vi "LDA_IP_DataTranslation.vi"() -> ()   [LabVIEW 2011]
uses:
  Globals/Meas_global.vi
  Data_Translation/DataTranslation_global.vi
  Globals/LDA_meas_global_1.vi
  PWA/PWAtasksGLOBAL.vi
  <userlib>/LV-Link3/PolySubVIs/DtCreateAinChan.vi
  <userlib>/LV-Link3/PolySubVIs/DtOLTimingSetInput.vi
  <userlib>/LV-Link3/PolySubVIs/DtOLTriggerDigital.vi
  Globals/LDA_meas_global_2.vi
  <userlib>/LV-Link3/PolySubVIs/DtOLReadMultiple2D.vi
panel:
  out "error out":errorcluster
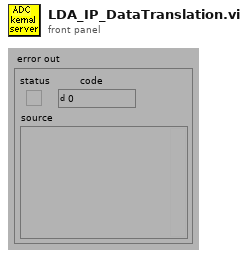
[diagram p1: front panel]
types:
  T1 = typedef "Ch_and_Spans.ctl" = cluster{"high limit (10V)":sgl, "low limit (-10V)":sgl, "Ch No":i16, "Var name":string, "Use Latest Calib":bool}
  T2 = typedef "Trigger_Mode.ctl" = enum16{"Free Running", "Start on Trigger", "Trigger Every Block", "Trigger Every Sample"}
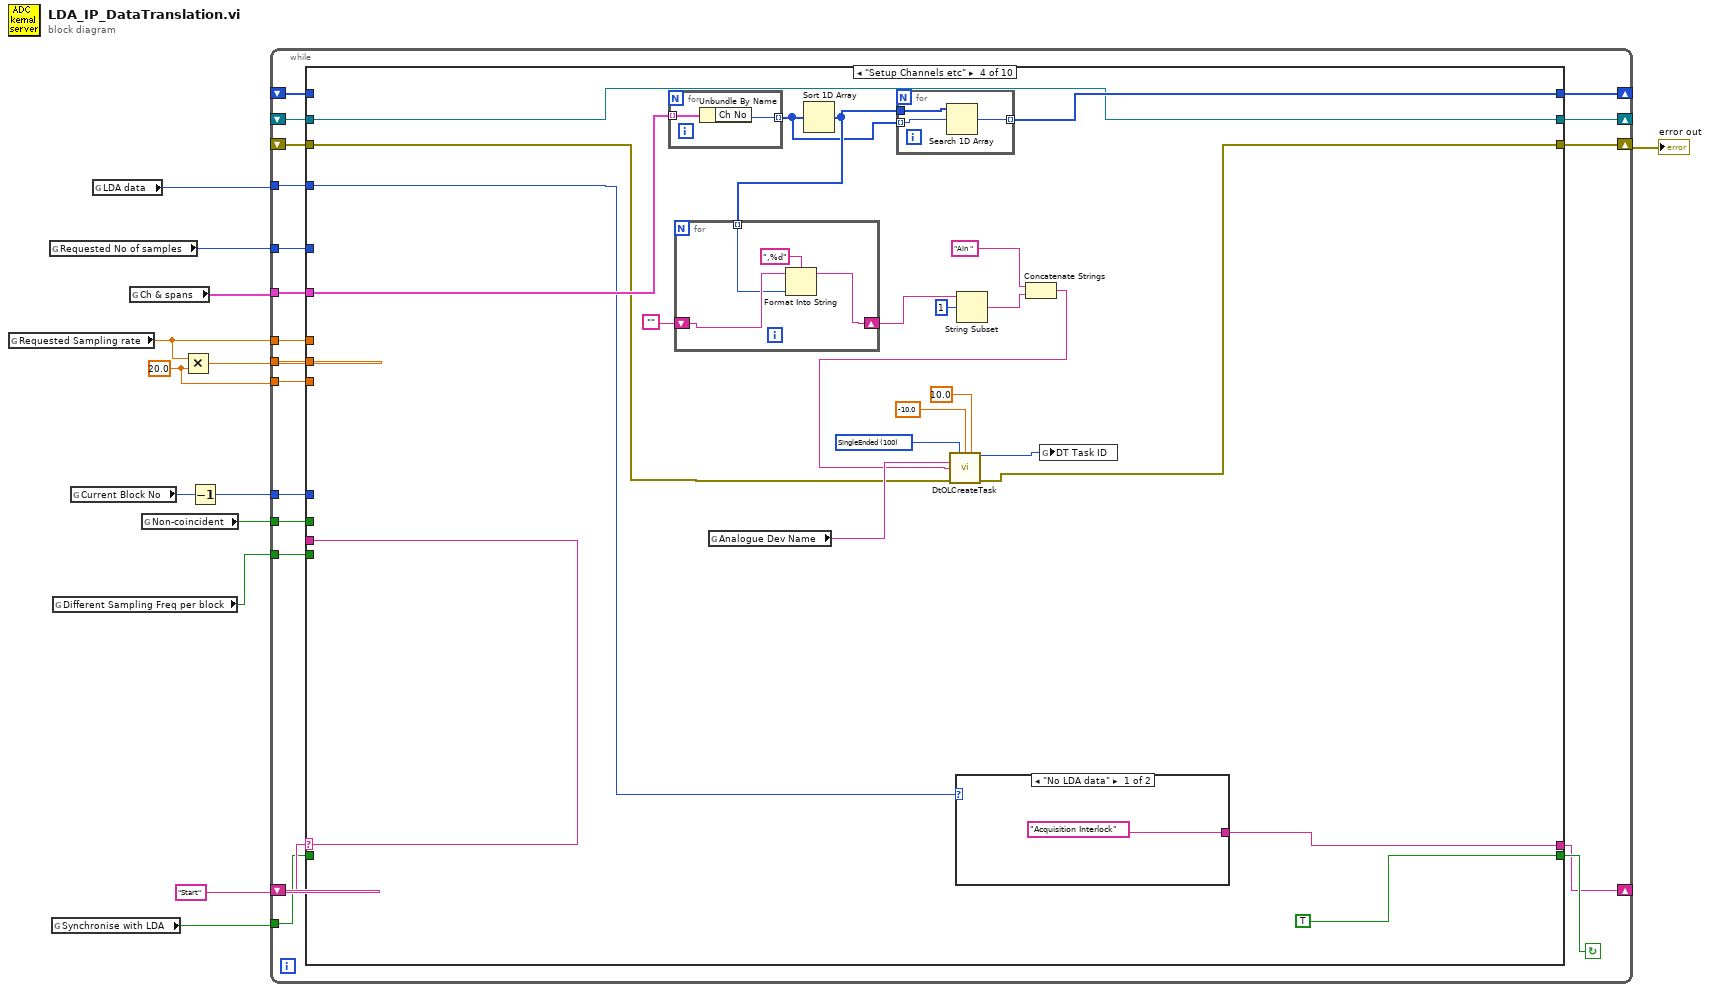
[diagram p0: block diagram]
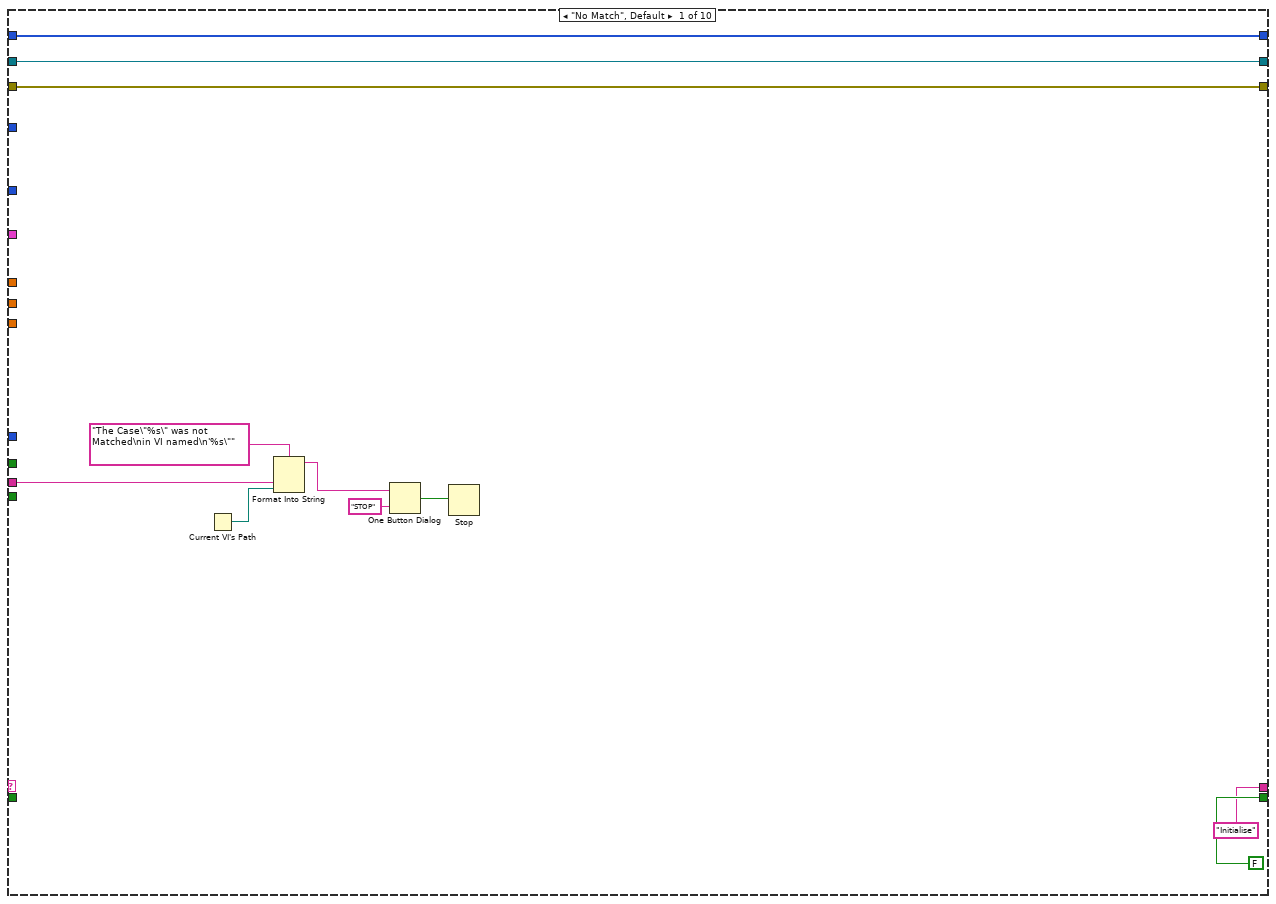
[diagram p2: hidden frame]
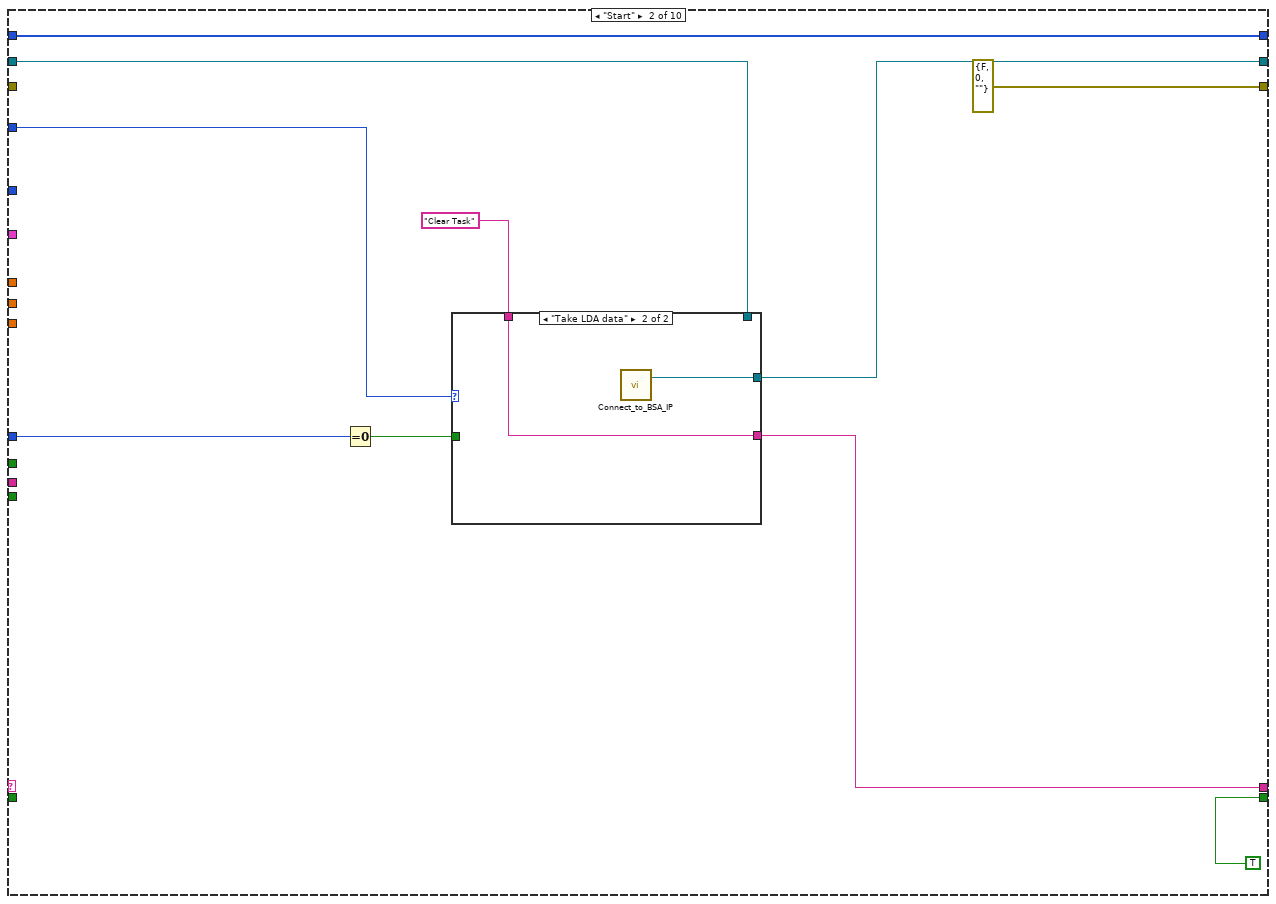
[diagram p3: hidden frame]
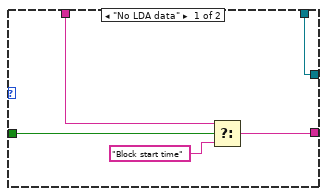
[diagram p4: hidden frame]
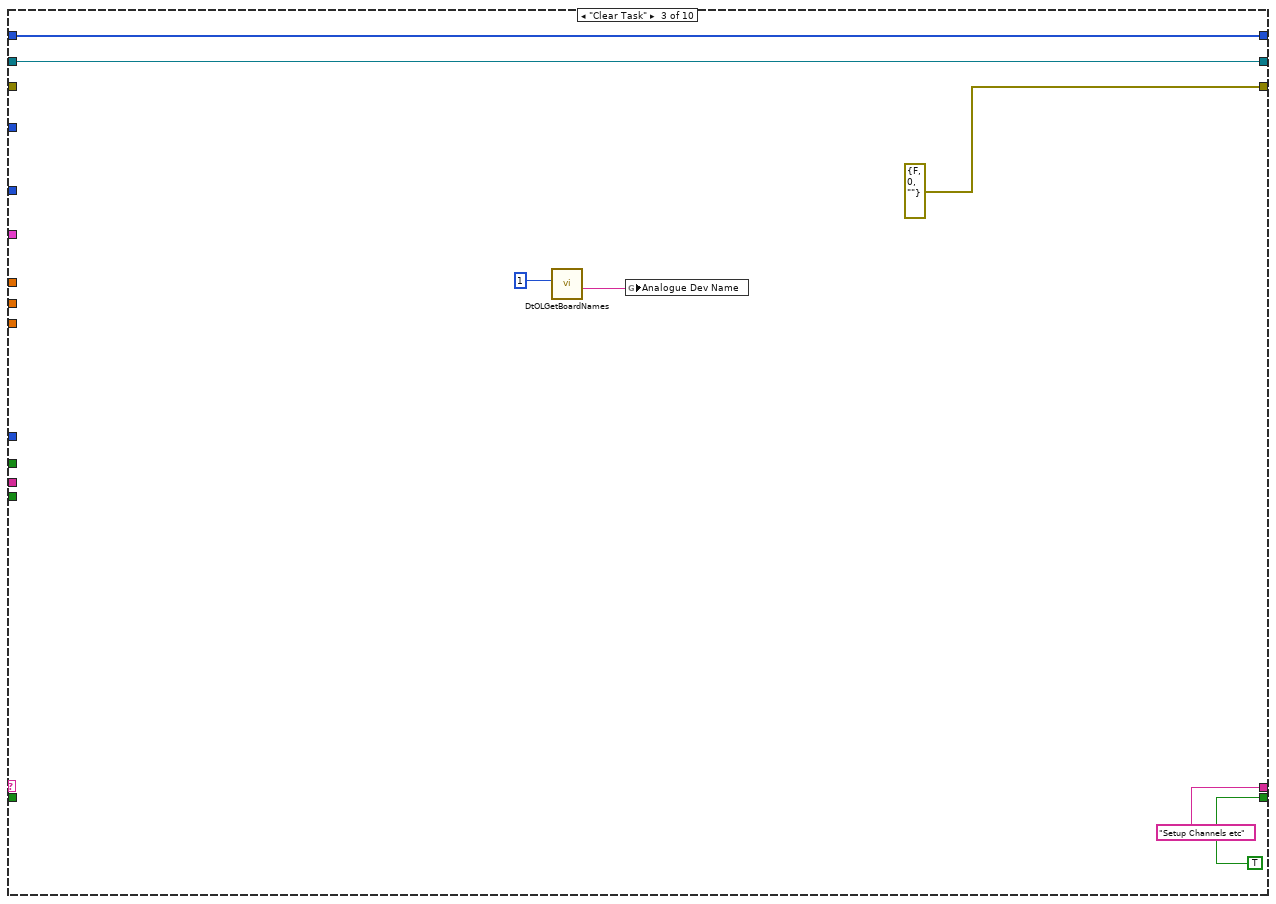
[diagram p5: hidden frame]
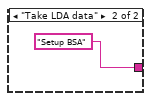
[diagram p6: hidden frame]
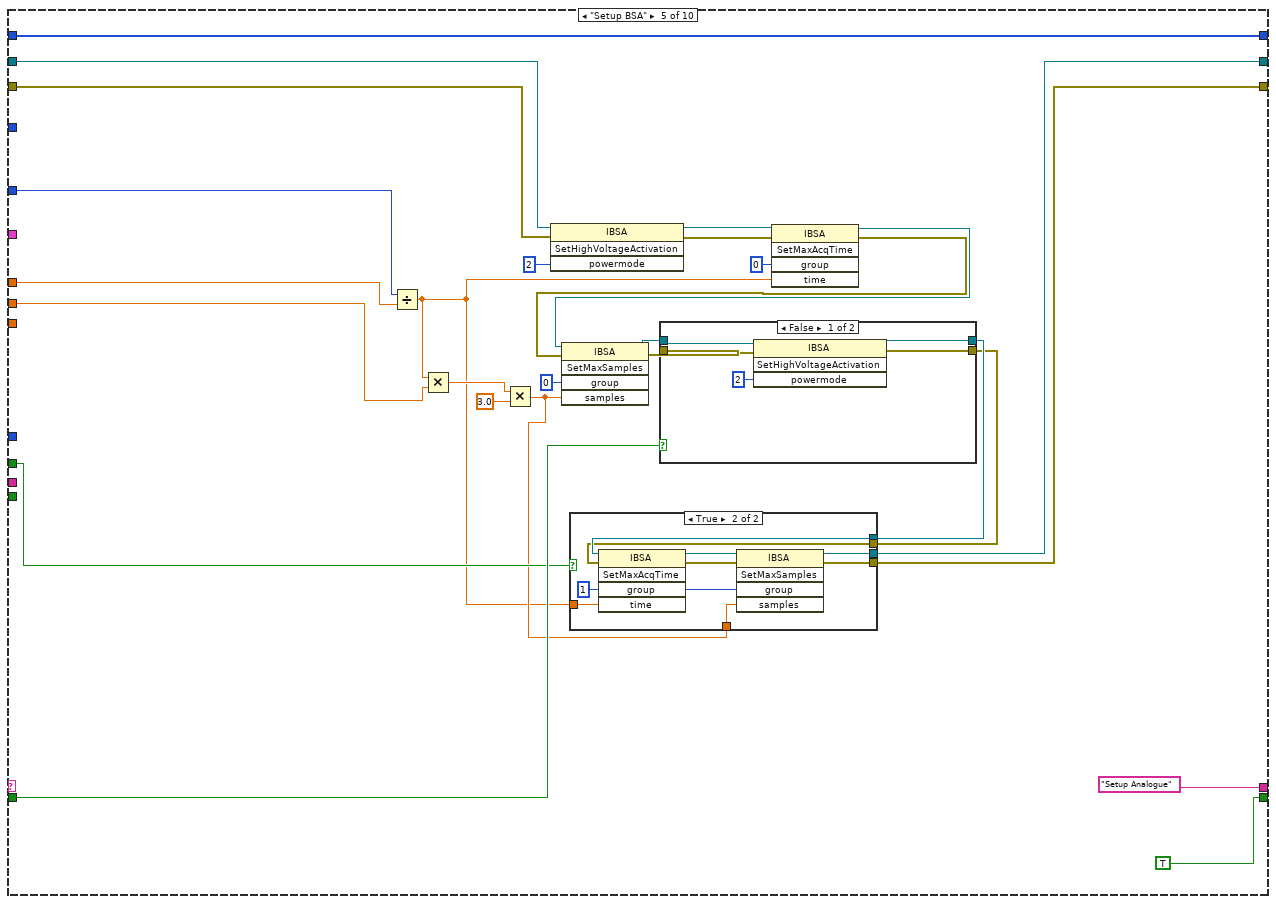
[diagram p7: hidden frame]
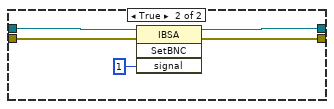
[diagram p9: hidden frame]
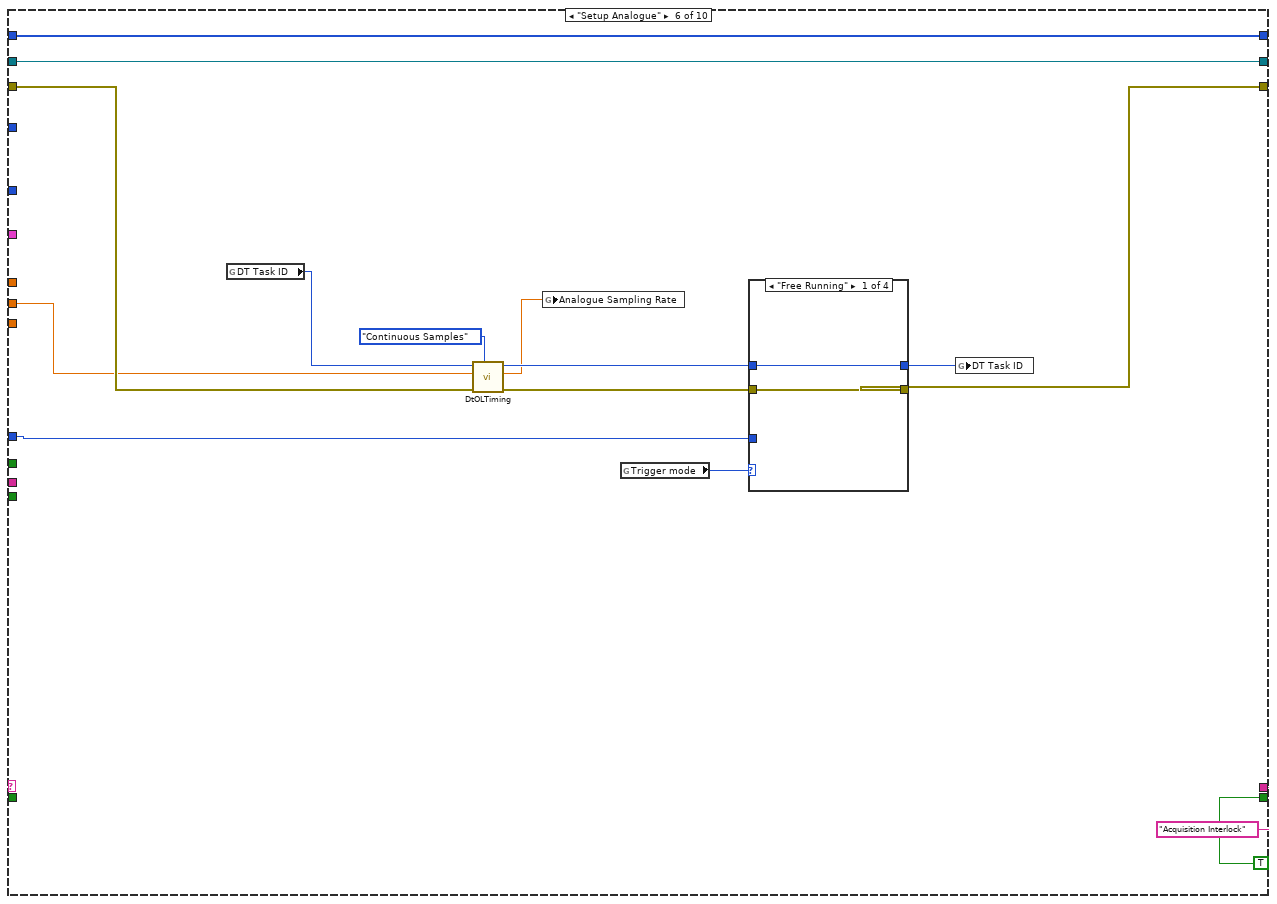
[diagram p10: hidden frame]
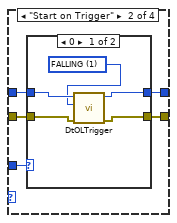
[diagram p11: hidden frame]
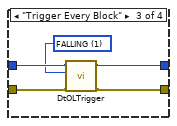
[diagram p13: hidden frame]
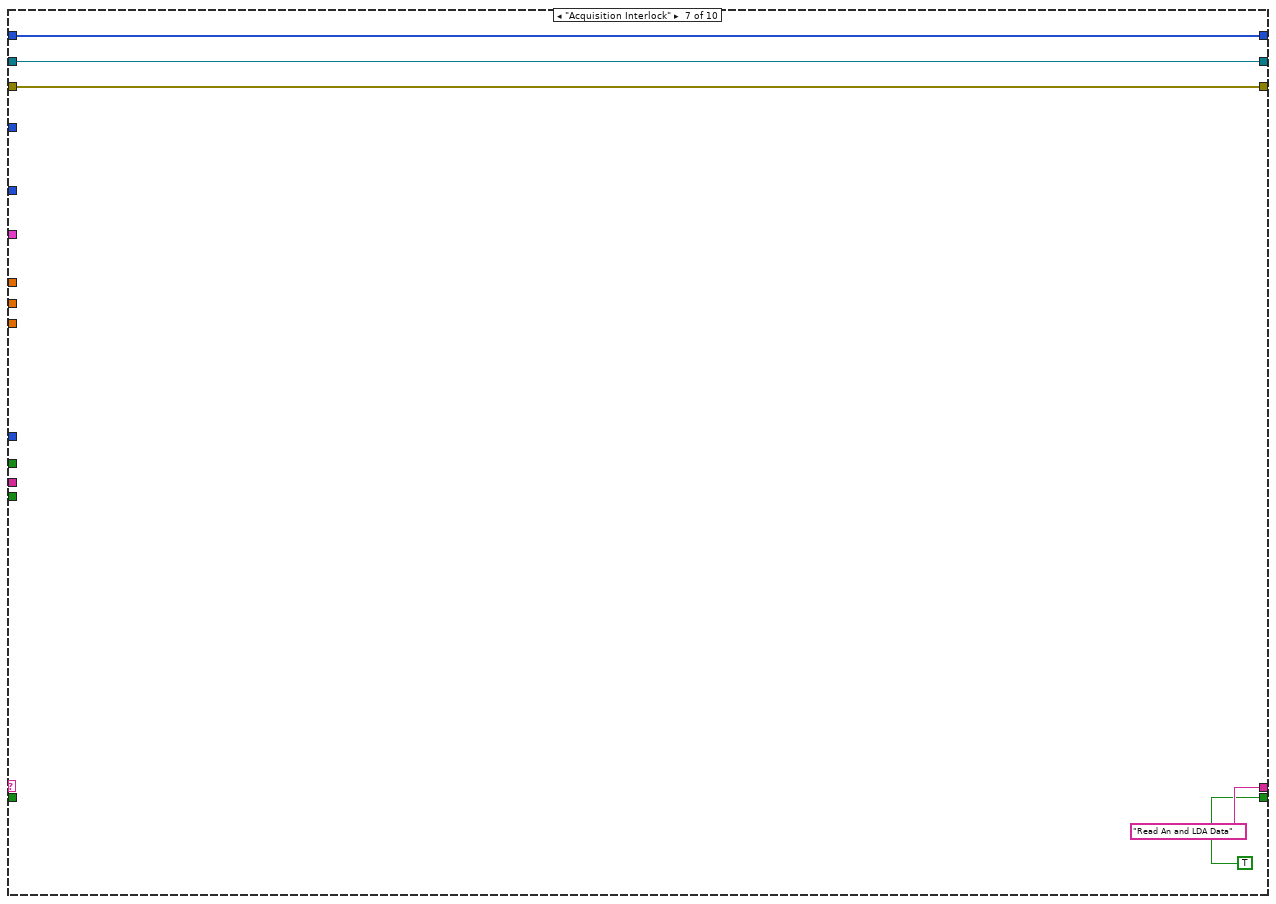
[diagram p15: hidden frame]
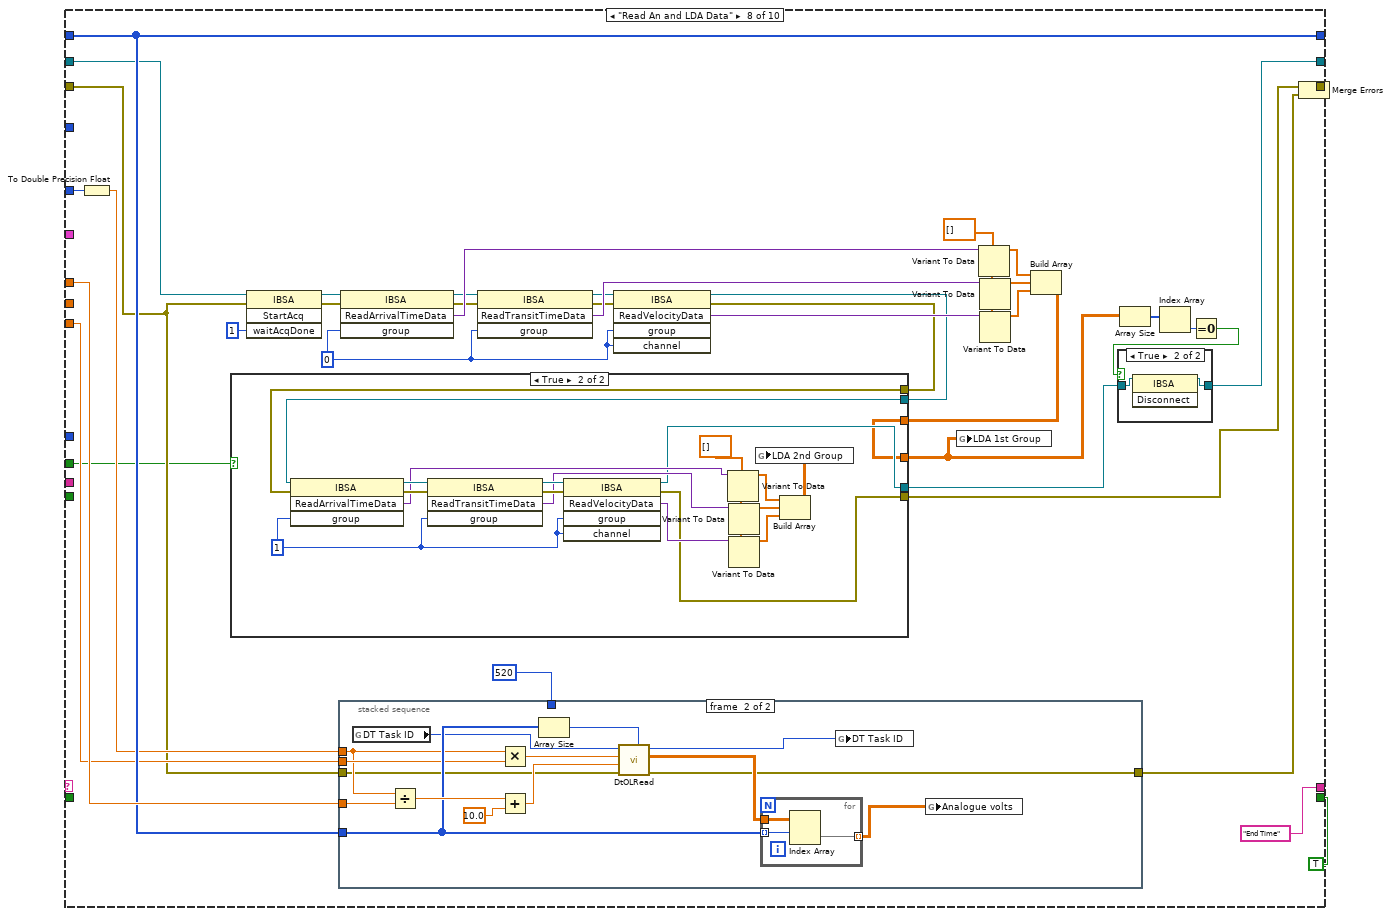
[diagram p16: hidden frame]
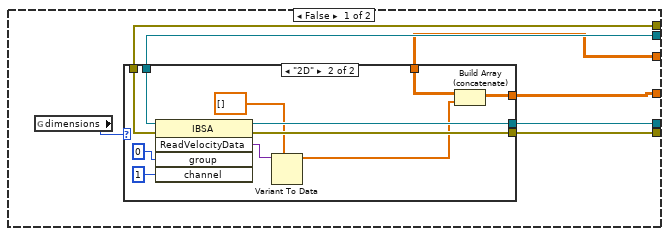
[diagram p17: hidden frame]
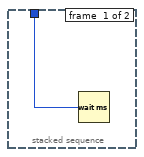
[diagram p20: hidden frame]
diagram:
  w8 = 20.0 ("y")
  n1 = global read "Meas_global.vi" "Requested Sampling rate"() -> (w2:dbl)
  n2 = global read "Meas_global.vi" "Requested No of samples"() -> (w1:i32)
  n3 = global read "Meas_global.vi" "Synchronise with LDA"() -> (w10:bool)
  n4 = global read "DataTranslation_global.vi" "Different Sampling Freq per block"() -> (w7:bool)
  n5 = global read "Meas_global.vi" "Current Block No"() -> (w5:i32)
  n6 = global read "Meas_global.vi" "LDA data"() -> (w11:enum16{"No LDA data", "Take LDA data"})
  n7 = global read "Meas_global.vi" "Ch & spans"() -> (w3:T1[])
  n8 = global read "LDA_meas_global_1.vi" "Non-coincident"() -> (w6:bool)
  n9 = Multiply(x=w2, y=w8) -> (x*y=w9:dbl)
  n10 = Decrement(x=w5) -> (x-1=w4:i32)
  n11 = while {
    shift-left: "Start" -> [w30]
    shift-right: [w31] -> _
    shift-right: [w24] -> w12
    shift-left: _ -> [w29]
    tunnel: w2 -> [w28]
    tunnel: w1 -> [w27]
    tunnel: w4 -> [w26]
    tunnel: w3 -> [w25]
    shift-right: [w23] -> _
    shift-left: _ -> [w22]
    tunnel: w11 -> [w21]
    shift-right: [w20] -> _
    shift-left: _ -> [w19]
    tunnel: w10 -> [w18]
    tunnel: w9 -> [w17]
    tunnel: w8 -> [w16]
    tunnel: w7 -> [w15]
    tunnel: w6 -> [w14]
    stop <- w32 continue-if-true
    n12 = case shown="\"Setup Channels etc\"" w30 {
      tunnel: [FALSE TRUE TRUE TRUE TRUE TRUE TRUE TRUE FALSE FALSE] -> w32
      tunnel: ["Initialise" w50 "Setup Channels etc" w88 "Setup Analogue" "Acquisition Interlock" "Read An and LDA Data" "End Time" "End" ("f") "End" ("f")] -> w31
      tunnel: w30 -> [w38 _ _ _ _ _ _ _ _ _]
      tunnel: [w35 errorcluster {"status"=FALSE, "code"=0, "source"=""} ("error out") errorcluster {"status"=FALSE, "code"=0, "source"=""} ("error out") w68 w100 w152 w187 w221 w296 w309] -> w24
      tunnel: w29 -> [w35 _ _ w69 w116 w159 w187 w214 w297 w309]
      tunnel: w28 -> [_ _ _ _ w113 _ _ w224 _ _]
      tunnel: w27 -> [_ _ _ _ w115 _ _ w217 _ _]
      tunnel: w26 -> [_ w52 _ _ _ w155 _ _ _ _]
      tunnel: w25 -> [_ _ _ w81 _ _ _ _ _ _]
      tunnel: [w34 w48 w65 w78 w112 w154 w185 w219 w300 w308] -> w23
      tunnel: w22 -> [w34 w48 w65 _ w112 w154 w185 w219 w300 w308]
      tunnel: w21 -> [_ w47 _ w76 _ _ _ _ w291 _]
      tunnel: [w33 w45 w64 w77 w101 w162 w184 w220 w299 w307] -> w20
      tunnel: w19 -> [w33 w44 w64 w77 w117 w162 w184 w215 w299 w307]
      tunnel: w18 -> [_ _ _ _ w114 _ _ _ _ _]
      tunnel: w17 -> [_ _ _ _ w109 w157 _ _ _ _]
      tunnel: w16 -> [_ _ _ _ _ _ _ w218 _ _]
      tunnel: w15 -> [_ _ _ _ _ _ _ _ _ _]
      tunnel: w14 -> [_ _ _ _ w108 _ _ w213 _ _]
      frame "No Match", Default {
        n13 = Current VI's Path() -> (path=w37:path)
        n14 = Format Into String(format string="The Case\"%s\" was not Matched\nin VI named\n'%s\"" ("Format String"), w38, w37) -> (resulting string=w41:string)  [unwired: 2 in, 1 out]
        n15 = One Button Dialog(message=w41, button name ("OK")="STOP") -> (true=w39:bool)
        n16 = Stop(stop? (T)=w39) -> ()
      }
      frame "Start" {
        n17 = Equal To 0?(x=w52) -> (x = 0?=w51:bool)
        n18 = case shown="\"Take LDA data\"" w47 {
          tunnel: w51 -> [w57 _]
          tunnel: [w56 w60] -> w50
          tunnel: "Clear Task" -> [w55 w60]
          tunnel: [w54 w59] -> w45
          tunnel: w44 -> [w54 _]
          frame "No LDA data" {
            n19 = Select(t=w55, s=w57, f="Block start time") -> (s? t:f=w56:string)
          }
          frame "Take LDA data" {
            n20 = call "Connect_to_BSA_IP.vi"() -> ("BSA"=w59:refnum<k7>)  [unwired: 3 out]
          }
        }
      }
      frame "Clear Task" {
        n21 = call <userlib>:"DtOLGetBoardNames.vi"("Select Board"=u32 1) -> ("Board Name"=w61:string)  [unwired: 8 in, 2 out]
        n22 = global write "PWAtasksGLOBAL.vi" "Analogue Dev Name"(w61) -> ()
      }
      frame "Setup Channels etc" {
        w73 = 100 items=["SingleEnded"=100, "Differential"=101] ("Channel Type")
        n23 = for {
          tunnel: w81 -> [w95] mode=indexing
          tunnel: [w94] -> w79 mode=indexing
          n24 = Unbundle By Name(w95) -> ("Ch No"=w94:i16)
        }
        n25 = global read "PWAtasksGLOBAL.vi" "Analogue Dev Name"() -> (w71:string)
        n26 = Sort 1D Array(array=w79) -> (sorted array=w80:i16[])
        n27 = for {
          shift-right: [w97] -> w86
          shift-left: "" -> [w98]
          tunnel: w80 -> [w96] mode=indexing
          n28 = Format Into String(format string=",%d", initial string=w98, w96) -> (resulting string=w97:string)  [unwired: 1 in, 1 out]
        }
        n29 = for {
          tunnel: w80 -> [w93]
          tunnel: w79 -> [w92] mode=indexing
          tunnel: [w91] -> w78 mode=indexing
          n30 = Search 1D Array(1D array=w93, element=w92) -> (index of element=w91:i32)  [unwired: 1 in]
        }
        n31 = case shown="\"No LDA data\"" w76 {
          tunnel: ["Acquisition Interlock" "Setup BSA"] -> w88
          frame "No LDA data" {
          }
          frame "Take LDA data" {
          }
        }
        n32 = String Subset(string=w86, offset (0)=1) -> (substring=w83:string)  [unwired: 1 in]
        n33 = Concatenate Strings("Ain ", w83) -> (w70:string)
        n34 = call-poly <userlib>:"DtOLCreateTask.vi"("Channel Type"=w73, "Range Min"=-10.0, "Range Max"=10.0, "Board Name"=w71, "Channel"=w70, "error in (no error)"=w69) -> ("Task out"=w72:i32, "error out"=w68:errorcluster)  [unwired: 7 in, 1 out]
        n35 = global write "DataTranslation_global.vi" "DT Task ID"(w72) -> ()
      }
      frame "Setup BSA" {
        n36 = Divide(x=w115, y=w113) -> (x/y=w104:dbl)
        n37 = Multiply(x=w104, y=w109) -> (x*y=w124:dbl)
        n38 = Multiply(x=w124, y=3.0) -> (x*y=w105:dbl)
        n39 = invoke class="IBSA" method="SetHighVoltageActivation"(reference=w117, error in=w116, "powermode"=2) -> (reference out=w119:refnum<k7>, error out=w118:errorcluster)  [unwired: 1 in, 2 out]
        n40 = invoke class="IBSA" method="SetMaxAcqTime"(reference=w119, error in=w118, "group"=0, "time"=w104) -> (reference out=w106:refnum<k7>, error out=w107:errorcluster)  [unwired: 1 in, 3 out]
        n41 = invoke class="IBSA" method="SetMaxSamples"(reference=w106, error in=w107, "group"=0, "samples"=w105) -> (reference out=w125:refnum<k7>, error out=w126:errorcluster)  [unwired: 1 in, 3 out]
        n42 = case shown="False" w114 {
          tunnel: w125 -> [w141 w144]
          tunnel: w126 -> [w140 w146]
          tunnel: [w139 w143] -> w103
          tunnel: [w138 w145] -> w102
          frame False {
            n43 = invoke class="IBSA" method="SetHighVoltageActivation"(reference=w141, error in=w140, "powermode"=2) -> (reference out=w139:refnum<k7>, error out=w138:errorcluster)  [unwired: 1 in, 2 out]
          }
          frame True {
            n44 = invoke class="IBSA" method="SetBNC"(reference=w144, error in=w146, "signal"=1) -> (reference out=w143:refnum<k7>, error out=w145:errorcluster)  [unwired: 1 in, 2 out]
          }
        }
        n45 = case shown="True" w108 {
          tunnel: w103 -> [w128 w135]
          tunnel: [w128 w133] -> w101
          tunnel: w102 -> [w127 w132]
          tunnel: [w127 w131] -> w100
          tunnel: w104 -> [_ w130]
          tunnel: w105 -> [_ w129]
          frame False {
          }
          frame True {
            w136 = 1 ("group")
            n46 = invoke class="IBSA" method="SetMaxAcqTime"(reference=w135, error in=w132, "group"=w136, "time"=w130) -> (reference out=w134:refnum<k7>, error out=w137:errorcluster)  [unwired: 1 in, 3 out]
            n47 = invoke class="IBSA" method="SetMaxSamples"(reference=w134, error in=w137, "group"=w136, "samples"=w129) -> (reference out=w133:refnum<k7>, error out=w131:errorcluster)  [unwired: 1 in, 3 out]
          }
        }
      }
      frame "Setup Analogue" {
        n48 = global read "DataTranslation_global.vi" "DT Task ID"() -> (w161:i32)
        n49 = call-poly <userlib>:"DtOLTiming.vi"("Sample Mode"=enum16{"Finite Samples", "Continuous Samples"}."Continuous Samples", "error in (no error)"=w159, "Sample Freq (Hz)"=w157, "Task in"=w161) -> ("error out"=w158:errorcluster, "Actual Sample Freq"=w148:dbl, "Task out"=w156:i32)  [unwired: 4 in, 1 out]
        n50 = global write "Meas_global.vi" "Analogue Sampling Rate"(w148) -> ()
        n51 = global read "Meas_global.vi" "Trigger mode"() -> (w149:T2)
        n52 = case shown="\"Free Running\"" w149 {
          tunnel: [w164 w166 w180 w183] -> w153
          tunnel: w156 -> [w164 w168 w181 w183]
          tunnel: [w163 w165 w177 w182] -> w152
          tunnel: w158 -> [w163 w167 w178 w182]
          tunnel: w155 -> [_ w169 _ _]
          frame "Free Running" {
          }
          frame "Start on Trigger" {
            n53 = case shown="0" w169 {
              tunnel: w168 -> [w174 w176]
              tunnel: w167 -> [w172 w175]
              tunnel: [w170 w176] -> w166
              tunnel: [w171 w175] -> w165
              frame 0 {
                w173 = 1 items=["RISING", "FALLING"] ("External Trigger Polarity")
                n54 = call-poly <userlib>:"DtOLTrigger.vi"("error in (no error)"=w172, "External Trigger Polarity"=w173, "Task in"=w174) -> ("error out"=w171:errorcluster, "Task out"=w170:i32)  [unwired: 7 in]
              }
              frame 1, Default {
              }
            }
          }
          frame "Trigger Every Block" {
            w179 = 1 items=["RISING", "FALLING"] ("External Trigger Polarity")
            n55 = call-poly <userlib>:"DtOLTrigger.vi"("error in (no error)"=w178, "External Trigger Polarity"=w179, "Task in"=w181) -> ("error out"=w177:errorcluster, "Task out"=w180:i32)  [unwired: 7 in]
          }
          frame "Trigger Every Sample" {
          }
        }
        n56 = global write "DataTranslation_global.vi" "DT Task ID"(w153) -> ()
      }
      frame "Acquisition Interlock" {
      }
      frame "Read An and LDA Data" {
        w203 = dbl[] [] ("Array Constant")
        w198 = 0 ("group")
        n57 = To Double Precision Float(number=w217) -> (double precision float=w216:dbl)
        n58 = invoke class="IBSA" method="StartAcq"(reference=w215, error in=w214, "waitAcqDone"=1) -> (reference out=w195:refnum<k7>, error out=w196:errorcluster)  [unwired: 1 in, 2 out]
        n59 = stacked-sequence {
          tunnel: w224 -> [_ w278]
          tunnel: [_ w272] -> w222
          tunnel: w219 -> [_ w277]
          tunnel: w218 -> [_ w276]
          tunnel: w216 -> [_ w275]
          tunnel: w214 -> [_ w274]
          tunnel: u32 520 -> [w269 _]
          frame #0 {
            n60 = Wait (ms)(milliseconds to wait=w269) -> ()  [unwired: 1 out]
          }
          frame #1 {
            n61 = global read "DataTranslation_global.vi" "DT Task ID"() -> (w273:i32)
            n62 = Divide(x=w275, y=w278) -> (x/y=w281:dbl)
            n63 = Multiply(x=w275, y=w276) -> (x*y=w280:dbl)
            n64 = Add(x=w281, y=10.0) -> (x+y=w283:dbl)
            n65 = Array Size(array=w277) -> (size(s)=w279:i32)
            n66 = call-poly <userlib>:"DtOLRead.vi"("Number Chan to Read"=w279, "error in (no error)"=w274, "Timeout"=w283, "Samples Per Channel"=w280, "Task in"=w273) -> ("error out"=w272:errorcluster, "2D Data out"=w284:dbl[][], "Task out"=w271:i32)  [unwired: 2 in, 2 out]
            n67 = for {
              tunnel: w277 -> [w287] mode=indexing
              tunnel: w284 -> [w286]
              tunnel: [w285] -> w270 mode=indexing
              n68 = Index Array(array=w286, index (row)=w287) -> (element=w285:dbl[])  [unwired: 1 in]
            }
            n69 = global write "DataTranslation_global.vi" "DT Task ID"(w271) -> ()
            n70 = global write "Meas_global.vi" "Analogue volts"(w270) -> ()
          }
        }
        n71 = invoke class="IBSA" method="ReadArrivalTimeData"(reference=w195, error in=w196, "group"=w198) -> (reference out=w199:refnum<k7>, error out=w200:errorcluster, "ReadArrivalTimeData"=w204:variant)  [unwired: 1 in, 1 out]
        n72 = invoke class="IBSA" method="ReadTransitTimeData"(reference=w199, error in=w200, "group"=w198) -> (reference out=w201:refnum<k7>, error out=w202:errorcluster, "ReadTransitTimeData"=w205:variant)  [unwired: 1 in, 1 out]
        n73 = invoke class="IBSA" method="ReadVelocityData"(reference=w201, error in=w202, "group"=w198, "channel"=w198) -> (reference out=w193:refnum<k7>, error out=w194:errorcluster, "ReadVelocityData"=w206:variant)  [unwired: 1 in, 2 out]
        n74 = Variant To Data(type=w203, Variant=w204) -> (data=w207:dbl[])  [unwired: 1 in, 1 out]
        n75 = Variant To Data(type=w203, Variant=w205) -> (data=w208:dbl[])  [unwired: 1 in, 1 out]
        n76 = Variant To Data(type=w203, Variant=w206) -> (data=w209:dbl[])  [unwired: 1 in, 1 out]
        n77 = Build Array(w207, w208, w209) -> (w191:dbl[][])
        n78 = case shown="True" w213 {
          tunnel: w194 -> [w232 w260]
          tunnel: w193 -> [w231 w259]
          tunnel: [w230 w250] -> w223
          tunnel: [w229 w249] -> w192
          tunnel: w191 -> [w227 w248]
          tunnel: [w228 w248] -> w190
          frame False {
            n79 = global read "Meas_global.vi" "dimensions"() -> (w233:enum16{"1D", "2D"})
            n80 = case shown="\"2D\"" w233 {
              tunnel: [w236 w245] -> w229
              tunnel: w231 -> [w236 w244]
              tunnel: w232 -> [w235 w243]
              tunnel: [w235 w242] -> w230
              tunnel: [w234 w238] -> w228
              tunnel: w227 -> [w234 w239]
              frame "1D" {
              }
              frame "2D" {
                n81 = invoke class="IBSA" method="ReadVelocityData"(reference=w244, error in=w243, "group"=0, "channel"=1) -> (reference out=w245:refnum<k7>, error out=w242:errorcluster, "ReadVelocityData"=w246:variant)  [unwired: 1 in, 2 out]
                n82 = Variant To Data(type=dbl[] [] ("Array Constant"), Variant=w246) -> (data=w237:dbl[])  [unwired: 1 in, 1 out]
                n83 = Build Array (concatenate)(w239, w237) -> (w238:dbl[][])
              }
            }
          }
          frame True {
            w254 = dbl[] [] ("Array Constant")
            w265 = 1 ("group")
            n84 = invoke class="IBSA" method="ReadArrivalTimeData"(reference=w259, error in=w260, "group"=w265) -> (reference out=w264:refnum<k7>, error out=w263:errorcluster, "ReadArrivalTimeData"=w253:variant)  [unwired: 1 in, 1 out]
            n85 = invoke class="IBSA" method="ReadTransitTimeData"(reference=w264, error in=w263, "group"=w265) -> (reference out=w262:refnum<k7>, error out=w261:errorcluster, "ReadTransitTimeData"=w252:variant)  [unwired: 1 in, 1 out]
            n86 = invoke class="IBSA" method="ReadVelocityData"(reference=w262, error in=w261, "group"=w265, "channel"=w265) -> (reference out=w249:refnum<k7>, error out=w250:errorcluster, "ReadVelocityData"=w251:variant)  [unwired: 1 in, 2 out]
            n87 = Variant To Data(type=w254, Variant=w253) -> (data=w258:dbl[])  [unwired: 1 in, 1 out]
            n88 = Variant To Data(type=w254, Variant=w252) -> (data=w257:dbl[])  [unwired: 1 in, 1 out]
            n89 = Variant To Data(type=w254, Variant=w251) -> (data=w256:dbl[])  [unwired: 1 in, 1 out]
            n90 = Build Array(w258, w257, w256) -> (w255:dbl[][])
            n91 = global write "LDA_meas_global_2.vi" "LDA 2nd Group"(w255) -> ()
          }
        }
        n92 = global write "LDA_meas_global_2.vi" "LDA 1st Group"(w190) -> ()
        n93 = Array Size(array=w190) -> (size(s)=w210:i32[])
        n94 = Index Array(array=w210) -> (element=w211:i32)  [unwired: 1 in]
        n95 = Equal To 0?(x=w211) -> (x = 0?=w212:bool)
        n96 = case shown="True" w212 {
          tunnel: w192 -> [w266 w268]
          tunnel: [w266 w267] -> w220
          frame False {
          }
          frame True {
            n97 = invoke class="IBSA" method="Disconnect"(reference=w268) -> (reference out=w267:refnum<k7>)  [unwired: 2 in, 2 out]
          }
        }
        n98 = Merge Errors(w223, w222) -> (w221:errorcluster)
      }
      frame "End Time" {
        n99 = Equal?(x=w291, y=enum16{"No LDA data", "Take LDA data"}."Take LDA data" ("LDA data")) -> (x = y?=w290:bool)
        n100 = global read "Meas_global.vi" "Requested No of blocks"() -> (w294:i32)
        n101 = global read "Meas_global.vi" "Current Block No"() -> (w295:i32)
        n102 = Increment(x=w295) -> (x+1=w293:i32)
        n103 = global read "DataTranslation_global.vi" "DT Task ID"() -> (w298:i32)
        n104 = Equal?(x=w294, y=w293) -> (x = y?=w289:bool)
        n105 = Or(x=w290, y=w289) -> (x .or. y?=w288:bool)
        n106 = case shown="True" w288 {
          tunnel: w298 -> [_ w306]
          tunnel: w297 -> [w303 w305]
          tunnel: [w303 w304] -> w296
          frame False {
          }
          frame True {
            n107 = call <userlib>:"DtOLCloseTask.vi"("Error in"=w305, "Task in"=w306) -> ("Error Out"=w304:errorcluster)  [unwired: 9 in]
          }
        }
      }
      frame "Extra case" {
      }
    }
  }
  "error out" <- w12
